vi "输入数据解析.vi"(0 "单个参数补充":dbl, 1 "从板号":dbl=1.0, 2 "主板二维码":string="BNET01", 3 "从板二维码":string="BNET01", 5 "主板引用":refnum<vi>, 7 "从板引用":refnum<vi>, 9 "主板选项":string="三级故障阀值", 11 "枚举":enum16{"主板", "从板"}(ring), 12 "快换":bool caption="快换写入") -> (4 "输出数组":dbl[][](array[numeric]), 6 "数组长度":dbl[](array[numeric]), 8 "循环次数":i32, 10 "命令":u32, 14 "名称":string[](array[string]), 15 "命令序号":u32[](array[numeric]))   [LabVIEW 2013] (continued)
                }
                n4749 = Build Array(w12371, w12369) -> (w12372:i32[])
              }
            }
            n4750 = Insert Into Array(array=w12193, new element=w12194) -> (w12192:dbl[])  [unwired: 1 in]
          }
          n4751 = Build Array(w12189) -> (w12188:dbl[][])
          n4752 = Build Array("二级故障阀值") -> (w12179:string[])
        }
        frame "SOC过低(3)" {
          n4753 = Unbundle By Name(w12398) -> ("一级故障 3"=w12399:refnum<vi>)
          n4754 = property class="Clust (严格)"(reference=w12399) -> ("Value"=w12397:T4)  [unwired: 1 in, 2 out]
          n4755 = for {
            N: 17 -> [_]
            tunnel: w12397 -> [w12409]
            shift-right: [w12406] -> w12403
            shift-left: dbl[] [] -> [w12407]
            i -> [w12410]
            n4756 = case shown="12" w12410 {
              tunnel: w12409 -> [w12411 w12422 w12433 w12443 w12453 w12463 w12475 w12487 w12499 w12511 w12523 w12535 w12547 w12559 w12566 w12575 w12584]
              tunnel: [w12412 w12423 w12434 w12444 w12454 w12465 w12477 w12489 w12501 w12513 w12525 w12536 w12549 w12561 w12565 w12574 w12586] -> w12408
              frame 0, Default {
                # "总电压过高"
                n4757 = disable-structure shown="启用" {
                  disable-tunnel: [w12418 w12421] -> w12414
                  disable-tunnel: [w12417 w12421] -> w12413
                  disable-tunnel: w12411 -> [w12416 _]
                  frame Disabled {
                    n4758 = Unbundle By Name(w12416) -> ("总电压过高"=w12415:dbl)
                    n4759 = call "输入分辨率计算-EV05.vi"("1字节?"=FALSE, "数值"=w12415, "分辨率"=0.1) -> ("低字节"=w12418:dbl, "高字节1"=w12417:dbl)  [unwired: 2 in, 5 out]
                  }
                  frame Enabled {
                    w12421 = 255 ("高字节1")
                  }
                }
                n4760 = Build Array(w12413, w12414) -> (w12412:i32[])
              }
              frame 1 {
                # "总电压过低"
                n4761 = disable-structure shown="启用" {
                  disable-tunnel: [w12429 w12432] -> w12425
                  disable-tunnel: [w12428 w12432] -> w12424
                  disable-tunnel: w12422 -> [w12427 _]
                  frame Disabled {
                    n4762 = Unbundle By Name(w12427) -> ("总电压过低"=w12426:dbl)
                    n4763 = call "输入分辨率计算-EV05.vi"("1字节?"=FALSE, "数值"=w12426, "分辨率"=0.1) -> ("低字节"=w12429:dbl, "高字节1"=w12428:dbl)  [unwired: 2 in, 5 out]
                  }
                  frame Enabled {
                    w12432 = 255 ("高字节1")
                  }
                }
                n4764 = Build Array(w12424, w12425) -> (w12423:i32[])
              }
              frame 2 {
                # "温度过高"
                n4765 = disable-structure shown="启用" {
                  disable-tunnel: [w12439 255 ("高字节1")] -> w12435
                  disable-tunnel: w12433 -> [w12437 _]
                  frame Disabled {
                    n4766 = Unbundle By Name(w12437) -> ("温度过高"=w12436:dbl)
                    n4767 = call "输入分辨率计算-EV05.vi"("1字节?"=TRUE, "数值"=w12436, "偏移量"=-40.0, "分辨率"=1.0) -> ("高字节1"=w12439:dbl)  [unwired: 1 in, 6 out]
                  }
                  frame Enabled {
                  }
                }
                n4768 = Build Array(w12435) -> (w12434:i32[])
              }
              frame 3 {
                # "温度过低"
                n4769 = disable-structure shown="启用" {
                  disable-tunnel: [w12449 255 ("高字节1")] -> w12445
                  disable-tunnel: w12443 -> [w12447 _]
                  frame Disabled {
                    n4770 = Unbundle By Name(w12447) -> ("温度过低"=w12446:dbl)
                    n4771 = call "输入分辨率计算-EV05.vi"("1字节?"=TRUE, "数值"=w12446, "偏移量"=-40.0, "分辨率"=1.0) -> ("高字节1"=w12449:dbl)  [unwired: 1 in, 6 out]
                  }
                  frame Enabled {
                  }
                }
                n4772 = Build Array(w12445) -> (w12444:i32[])
              }
              frame 4 {
                # "整组温度不均衡"
                n4773 = disable-structure shown="启用" {
                  disable-tunnel: [w12459 255 ("高字节1")] -> w12455
                  disable-tunnel: w12453 -> [w12457 _]
                  frame Disabled {
                    n4774 = Unbundle By Name(w12457) -> ("整组温度不均衡"=w12456:dbl)
                    n4775 = call "输入分辨率计算-EV05.vi"("1字节?"=TRUE, "数值"=w12456, "偏移量"=0.0, "分辨率"=1.0) -> ("高字节1"=w12459:dbl)  [unwired: 1 in, 6 out]
                  }
                  frame Enabled {
                  }
                }
                n4776 = Build Array(w12455) -> (w12454:i32[])
              }
              frame 5 {
                # "单组电压不均衡"
                n4777 = disable-structure shown="启用" {
                  disable-tunnel: [w12471 w12474] -> w12466
                  disable-tunnel: [w12469 w12474] -> w12464
                  disable-tunnel: w12463 -> [w12468 _]
                  frame Disabled {
                    n4778 = Unbundle By Name(w12468) -> ("单组电压不均衡"=w12467:dbl)
                    n4779 = call "输入分辨率计算-EV05.vi"("1字节?"=FALSE, "数值"=w12467, "偏移量"=0.0, "分辨率"=0.001) -> ("低字节"=w12469:dbl, "高字节1"=w12471:dbl)  [unwired: 1 in, 5 out]
                  }
                  frame Enabled {
                    w12474 = 255 ("高字节1")
                  }
                }
                n4780 = Build Array(w12466, w12464) -> (w12465:i32[])
              }
              frame 6 {
                # "整组电压不均衡"
                n4781 = disable-structure shown="启用" {
                  disable-tunnel: [w12483 w12486] -> w12478
                  disable-tunnel: [w12481 w12486] -> w12476
                  disable-tunnel: w12475 -> [w12480 _]
                  frame Disabled {
                    n4782 = Unbundle By Name(w12480) -> ("整组电压不均衡"=w12479:dbl)
                    n4783 = call "输入分辨率计算-EV05.vi"("1字节?"=FALSE, "数值"=w12479, "偏移量"=0.0, "分辨率"=0.001) -> ("低字节"=w12481:dbl, "高字节1"=w12483:dbl)  [unwired: 1 in, 5 out]
                  }
                  frame Enabled {
                    w12486 = 255 ("高字节1")
                  }
                }
                n4784 = Build Array(w12478, w12476) -> (w12477:i32[])
              }
              frame 7 {
                # "单体电压过高"
                n4785 = disable-structure shown="启用" {
                  disable-tunnel: [w12495 w12498] -> w12490
                  disable-tunnel: [w12493 w12498] -> w12488
                  disable-tunnel: w12487 -> [w12492 _]
                  frame Disabled {
                    n4786 = Unbundle By Name(w12492) -> ("单体电压过高"=w12491:dbl)
                    n4787 = call "输入分辨率计算-EV05.vi"("1字节?"=FALSE, "数值"=w12491, "偏移量"=0.0, "分辨率"=0.001) -> ("低字节"=w12493:dbl, "高字节1"=w12495:dbl)  [unwired: 1 in, 5 out]
                  }
                  frame Enabled {
                    w12498 = 255 ("高字节1")
                  }
                }
                n4788 = Build Array(w12490, w12488) -> (w12489:i32[])
              }
              frame 8 {
                # "单体电压过低"
                n4789 = disable-structure shown="启用" {
                  disable-tunnel: [w12507 w12510] -> w12502
                  disable-tunnel: [w12505 w12510] -> w12500
                  disable-tunnel: w12499 -> [w12504 _]
                  frame Disabled {
                    n4790 = Unbundle By Name(w12504) -> ("单体电压过低"=w12503:dbl)
                    n4791 = call "输入分辨率计算-EV05.vi"("1字节?"=FALSE, "数值"=w12503, "偏移量"=0.0, "分辨率"=0.001) -> ("低字节"=w12505:dbl, "高字节1"=w12507:dbl)  [unwired: 1 in, 5 out]
                  }
                  frame Enabled {
                    w12510 = 255 ("高字节1")
                  }
                }
                n4792 = Build Array(w12502, w12500) -> (w12501:i32[])
              }
              frame 9 {
                # "充电电流过高"
                n4793 = disable-structure shown="启用" {
                  disable-tunnel: [w12519 w12522] -> w12514
                  disable-tunnel: [w12517 w12522] -> w12512
                  disable-tunnel: w12511 -> [w12516 _]
                  frame Disabled {
                    n4794 = Unbundle By Name(w12516) -> ("充电电流过高"=w12515:dbl)
                    n4795 = call "输入分辨率计算-EV05.vi"("1字节?"=FALSE, "数值"=w12515, "偏移量"=-3000.0, "分辨率"=0.1) -> ("低字节"=w12517:dbl, "高字节1"=w12519:dbl)  [unwired: 1 in, 5 out]
                  }
                  frame Enabled {
                    w12522 = 255 ("高字节1")
                  }
                }
                n4796 = Build Array(w12514, w12512) -> (w12513:i32[])
              }
              frame 10 {
                # "放电电流过高"
                n4797 = disable-structure shown="启用" {
                  disable-tunnel: [w12531 w12534] -> w12526
                  disable-tunnel: [w12529 w12534] -> w12524
                  disable-tunnel: w12523 -> [w12528 _]
                  frame Disabled {
                    n4798 = Unbundle By Name(w12528) -> ("放电电流过高"=w12527:dbl)
                    n4799 = call "输入分辨率计算-EV05.vi"("1字节?"=FALSE, "数值"=w12527, "偏移量"=-3000.0, "分辨率"=0.1) -> ("低字节"=w12529:dbl, "高字节1"=w12531:dbl)  [unwired: 1 in, 5 out]
                  }
                  frame Enabled {
                    w12534 = 255 ("高字节1")
                  }
                }
                n4800 = Build Array(w12526, w12524) -> (w12525:i32[])
              }
              frame 11 {
                # "单组温度不均衡"
                n4801 = disable-structure shown="启用" {
                  disable-tunnel: [w12541 255 ("高字节1")] -> w12537
                  disable-tunnel: w12535 -> [w12539 _]
                  frame Disabled {
                    n4802 = Unbundle By Name(w12539) -> ("单组温度不均衡"=w12538:dbl)
                    n4803 = call "输入分辨率计算-EV05.vi"("1字节?"=TRUE, "数值"=w12538, "偏移量"=0.0, "分辨率"=1.0) -> ("高字节1"=w12541:dbl)  [unwired: 1 in, 6 out]
                  }
                  frame Enabled {
                  }
                }
                n4804 = Build Array(w12537) -> (w12536:i32[])
              }
              frame 12 {
                # "SOC过高"
                n4805 = Unbundle By Name(w12547) -> ("SOC过高"=w12546:dbl)
                n4806 = call "输入分辨率计算-EV05.vi"("1字节?"=FALSE, "数值"=w12546, "偏移量"=0.0, "分辨率"=0.1) -> ()  [unwired: 1 in, 7 out]
                n4807 = disable-structure shown="启用" {
                  disable-tunnel: _ -> [w12553 _]
                  disable-tunnel: [w12553 255 ("高字节1")] -> w12545
                  disable-tunnel: [w12552 i32[] [] ("低位子数组")] -> _
                  disable-tunnel: _ -> [w12552 _]
                  frame Disabled {
                  }
                  frame Enabled {
                  }
                }
                n4808 = Build Array(w12545, w12545) -> (w12549:i32[])
              }
              frame 13 {
                n4809 = Unbundle By Name(w12559) -> ("SOC过低"=w12558:dbl)
                n4810 = call "输入分辨率计算-EV05.vi"("1字节?"=FALSE, "数值"=w12558, "偏移量"=0.0, "分辨率"=0.1) -> ("低字节"=w12556:dbl, "高字节1"=w12557:dbl)  [unwired: 1 in, 5 out]
                n4811 = Build Array(w12557, w12556) -> (w12561:dbl[])
              }
              frame 14 {
                # "内阻过大"
                n4812 = disable-structure shown="启用" {
                  disable-tunnel: w12566 -> [w12571 _]
                  disable-tunnel: [w12567 255 ("高字节1")] -> w12564
                  frame Disabled {
                    n4813 = Unbundle By Name(w12571) -> ("内阻过大"=w12570:dbl)
                    n4814 = call "输入分辨率计算-EV05.vi"("1字节?"=TRUE, "数值"=w12570, "分辨率"=0.1) -> ("高字节1"=w12567:dbl)  [unwired: 2 in, 6 out]
                  }
                  frame Enabled {
                  }
                }
                n4815 = Build Array(w12564) -> (w12565:i32[])
              }
              frame 15 {
                # "极柱温度过高"
                n4816 = disable-structure shown="启用" {
                  disable-tunnel: w12575 -> [w12581 _]
                  disable-tunnel: [w12577 255 ("高字节1")] -> w12573
                  frame Disabled {
                    n4817 = Unbundle By Name(w12581) -> ("极柱温度过高"=w12580:dbl)
                    n4818 = call "输入分辨率计算-EV05.vi"("1字节?"=TRUE, "数值"=w12580, "偏移量"=-40.0, "分辨率"=1.0) -> ("高字节1"=w12577:dbl)  [unwired: 1 in, 6 out]
                  }
                  frame Enabled {
                  }
                }
                n4819 = Build Array(w12573) -> (w12574:i32[])
              }
              frame 16 {
                # "SOH过低"
                n4820 = disable-structure shown="启用" {
                  disable-tunnel: [w12598 w12606] -> w12585
                  disable-tunnel: w12584 -> [w12595 _]
                  disable-tunnel: [w12587 w12606] -> w12583
                  frame Disabled {
                    n4821 = Unbundle By Name(w12595) -> ("SOH过低"=w12594:dbl)
                    n4822 = call "输入分辨率计算-EV05.vi"("1字节?"=FALSE, "数值"=w12594, "偏移量"=0.0, "分辨率"=0.1) -> ("低字节"=w12596:dbl, "高字节1"=w12597:dbl)  [unwired: 1 in, 5 out]
                    n4823 = call "二进制解析-8.6.vi"("索引"=4, "数值"=w12597) -> ("低位子数组"=w12600:i32[])  [unwired: 3 out]
                    n4824 = call "二进制解析-8.6.vi"("索引"=4, "数值"=w12596) -> ("低位子数组"=w12589:i32[], "高位子数组"=w12599:i32[])  [unwired: 2 out]
                    n4825 = call "二进制解析-8.6.vi"("索引"=4, "数值"=0) -> ("低位子数组"=w12590:i32[])  [unwired: 3 out]
                    n4826 = Insert Into Array(array=w12600, new element=w12599) -> (w12593:i32[])  [unwired: 1 in]
                    n4827 = Insert Into Array(array=w12589, new element=w12590) -> (w12588:i32[])  [unwired: 1 in]
                    n4828 = call "数值二进制转十进制-8.6.vi"("子数组"=w12593) -> ("十进制数值"=w12598:i32)  [unwired: 4 out]
                    n4829 = call "数值二进制转十进制-8.6.vi"("子数组"=w12588) -> ("十进制数值"=w12587:i32)  [unwired: 4 out]
                  }
                  frame Enabled {
                    w12606 = 255 ("高字节1")
                  }
                }
                n4830 = Build Array(w12585, w12583) -> (w12586:i32[])
              }
            }
            n4831 = Insert Into Array(array=w12407, new element=w12408) -> (w12406:dbl[])  [unwired: 1 in]
          }
          n4832 = Build Array(w12403) -> (w12402:dbl[][])
          n4833 = Build Array("三级故障阀值") -> (w12393:string[])
        }
        frame "二级故障阀值" {
          n4834 = Unbundle By Name(w12612) -> ("一级故障 2"=w12613:refnum<vi>)
          n4835 = property class="Clust (严格)"(reference=w12613) -> ("Value"=w12611:T4)  [unwired: 1 in, 2 out]
          n4836 = for {
            N: 17 -> [_]
            tunnel: w12611 -> [w12623]
            shift-right: [w12620] -> w12617
            shift-left: dbl[] [] -> [w12621]
            i -> [w12624]
            n4837 = case shown="4" w12624 {
              tunnel: w12623 -> [w12626 w12633 w12640 w12647 w12654 w12660 w12668 w12676 w12684 w12692 w12700 w12708 w12716 w12724 w12734 w12741 w12745]
              tunnel: [w12627 w12634 w12642 w12649 w12655 w12663 w12671 w12679 w12687 w12695 w12703 w12709 w12718 w12726 w12733 w12740 w12747] -> w12622
              frame 0, Default {
                # "总电压过高"
                n4838 = Unbundle By Name(w12626) -> ("总电压过高"=w12625:dbl)
                n4839 = call "输入分辨率计算-EV05.vi"("1字节?"=FALSE, "数值"=w12625, "分辨率"=0.1) -> ("低字节"=w12629:dbl, "高字节1"=w12628:dbl)  [unwired: 2 in, 5 out]
                n4840 = Build Array(w12628, w12629) -> (w12627:dbl[])
              }
              frame 1 {
                # "总电压过低"
                n4841 = Unbundle By Name(w12633) -> ("总电压过低"=w12632:dbl)
                n4842 = call "输入分辨率计算-EV05.vi"("1字节?"=FALSE, "数值"=w12632, "分辨率"=0.1) -> ("低字节"=w12636:dbl, "高字节1"=w12635:dbl)  [unwired: 2 in, 5 out]
                n4843 = Build Array(w12635, w12636) -> (w12634:dbl[])
              }
              frame 2 {
                # "温度过高"
                n4844 = Unbundle By Name(w12640) -> ("温度过高"=w12639:dbl)
                n4845 = call "输入分辨率计算-EV05.vi"("1字节?"=TRUE, "数值"=w12639, "偏移量"=-40.0, "分辨率"=1.0) -> ("高字节1"=w12643:dbl)  [unwired: 1 in, 6 out]
                n4846 = Build Array(w12643) -> (w12642:dbl[])
              }
              frame 3 {
                # "温度过低"
                n4847 = Unbundle By Name(w12647) -> ("温度过低"=w12646:dbl)
                n4848 = call "输入分辨率计算-EV05.vi"("1字节?"=TRUE, "数值"=w12646, "偏移量"=-40.0, "分辨率"=1.0) -> ("高字节1"=w12650:dbl)  [unwired: 1 in, 6 out]
                n4849 = Build Array(w12650) -> (w12649:dbl[])
              }
              frame 4 {
                # "整组温度不均衡"
                n4850 = Unbundle By Name(w12654) -> ("整组温度不均衡"=w12653:dbl)
                n4851 = call "输入分辨率计算-EV05.vi"("1字节?"=TRUE, "数值"=w12653, "分辨率"=1.0) -> ("高字节1"=w12656:dbl)  [unwired: 2 in, 6 out]
                n4852 = Build Array(w12656) -> (w12655:dbl[])
              }
              frame 5 {
                # "单组电压不均衡"
                n4853 = Unbundle By Name(w12660) -> ("单组电压不均衡"=w12659:dbl)
                n4854 = call "输入分辨率计算-EV05.vi"("1字节?"=FALSE, "数值"=w12659, "偏移量"=0.0, "分辨率"=0.001) -> ("低字节"=w12661:dbl, "高字节1"=w12664:dbl)  [unwired: 1 in, 5 out]
                n4855 = Build Array(w12664, w12661) -> (w12663:dbl[])
              }
              frame 6 {
                # "整组电压不均衡"
                n4856 = Unbundle By Name(w12668) -> ("整组电压不均衡"=w12667:dbl)
                n4857 = call "输入分辨率计算-EV05.vi"("1字节?"=FALSE, "数值"=w12667, "偏移量"=0.0, "分辨率"=0.001) -> ("低字节"=w12669:dbl, "高字节1"=w12672:dbl)  [unwired: 1 in, 5 out]
                n4858 = Build Array(w12672, w12669) -> (w12671:dbl[])
              }
              frame 7 {
                # "单体电压过高"
                n4859 = Unbundle By Name(w12676) -> ("单体电压过高"=w12675:dbl)
                n4860 = call "输入分辨率计算-EV05.vi"("1字节?"=FALSE, "数值"=w12675, "偏移量"=0.0, "分辨率"=0.001) -> ("低字节"=w12677:dbl, "高字节1"=w12680:dbl)  [unwired: 1 in, 5 out]
                n4861 = Build Array(w12680, w12677) -> (w12679:dbl[])
              }
              frame 8 {
                # "单体电压过低"
                n4862 = Unbundle By Name(w12684) -> ("单体电压过低"=w12683:dbl)
                n4863 = call "输入分辨率计算-EV05.vi"("1字节?"=FALSE, "数值"=w12683, "偏移量"=0.0, "分辨率"=0.001) -> ("低字节"=w12685:dbl, "高字节1"=w12688:dbl)  [unwired: 1 in, 5 out]
                n4864 = Build Array(w12688, w12685) -> (w12687:dbl[])
              }
              frame 9 {
                # "充电电流过高"
                n4865 = Unbundle By Name(w12692) -> ("充电电流过高"=w12691:dbl)
                n4866 = call "输入分辨率计算-EV05.vi"("1字节?"=FALSE, "数值"=w12691, "偏移量"=0.0, "分辨率"=0.1) -> ("低字节"=w12693:dbl, "高字节1"=w12696:dbl)  [unwired: 1 in, 5 out]
                n4867 = Build Array(w12696, w12693) -> (w12695:dbl[])
              }
              frame 10 {
                # "放电电流过高"
                n4868 = Unbundle By Name(w12700) -> ("放电电流过高"=w12699:dbl)
                n4869 = call "输入分辨率计算-EV05.vi"("1字节?"=FALSE, "数值"=w12699, "偏移量"=0.0, "分辨率"=0.1) -> ("低字节"=w12701:dbl, "高字节1"=w12704:dbl)  [unwired: 1 in, 5 out]
                n4870 = Build Array(w12704, w12701) -> (w12703:dbl[])
              }
              frame 11 {
                # "单组温度不均衡"
                n4871 = Unbundle By Name(w12708) -> ("单组温度不均衡"=w12707:dbl)
                n4872 = call "输入分辨率计算-EV05.vi"("1字节?"=TRUE, "数值"=w12707, "分辨率"=1.0) -> ("高字节1"=w12710:dbl)  [unwired: 2 in, 6 out]
                n4873 = Build Array(w12710) -> (w12709:dbl[])
              }
              frame 12 {
                # "SOC过高"
                n4874 = Unbundle By Name(w12716) -> ("SOC过高"=w12715:dbl)
                n4875 = call "输入分辨率计算-EV05.vi"("1字节?"=FALSE, "数值"=w12715, "偏移量"=0.0, "分辨率"=0.1) -> ("低字节"=w12713:dbl, "高字节1"=w12714:dbl)  [unwired: 1 in, 5 out]
                n4876 = Build Array(w12714, w12713) -> (w12718:dbl[])
              }
              frame 13 {
                # "SOC过低"
                n4877 = Unbundle By Name(w12724) -> ("SOC过低"=w12723:dbl)
                n4878 = call "输入分辨率计算-EV05.vi"("1字节?"=FALSE, "数值"=w12723, "偏移量"=0.0, "分辨率"=0.1) -> ("低字节"=w12721:dbl, "高字节1"=w12722:dbl)  [unwired: 1 in, 5 out]
                n4879 = Build Array(w12722, w12721) -> (w12726:dbl[])
              }
              frame 14 {
                # "内阻过大"
                n4880 = Unbundle By Name(w12734) -> ("内阻过大"=w12732:dbl)
                n4881 = call "输入分辨率计算-EV05.vi"("1字节?"=TRUE, "数值"=w12732, "分辨率"=0.1) -> ("高字节1"=w12729:dbl)  [unwired: 2 in, 6 out]
                n4882 = Build Array(w12729) -> (w12733:dbl[])
              }
              frame 15 {
                # "极柱温度过高"
                n4883 = Unbundle By Name(w12741) -> ("极柱温度过高"=w12739:dbl)
                n4884 = call "输入分辨率计算-EV05.vi"("1字节?"=TRUE, "数值"=w12739, "偏移量"=-40.0, "分辨率"=1.0) -> ("高字节1"=w12736:dbl)  [unwired: 1 in, 6 out]
                n4885 = Build Array(w12736) -> (w12740:dbl[])
              }
              frame 16 {
                # "SOH过低"
                n4886 = Unbundle By Name(w12745) -> ("SOH过低"=w12744:dbl)
                n4887 = call "输入分辨率计算-EV05.vi"("1字节?"=FALSE, "数值"=w12744, "偏移量"=0.0, "分辨率"=0.1) -> ("低字节"=w12742:dbl, "高字节1"=w12743:dbl)  [unwired: 1 in, 5 out]
                n4888 = Build Array(w12743, w12742) -> (w12747:dbl[])
              }
            }
            n4889 = Insert Into Array(array=w12621, new element=w12622) -> (w12620:dbl[])  [unwired: 1 in]
          }
          n4890 = Build Array(w12617) -> (w12616:dbl[][])
          n4891 = Build Array("二级故障阀值") -> (w12607:string[])
        }
        frame "三级故障阀值" {
          n4892 = Unbundle By Name(w12755) -> ("一级故障 3"=w12756:refnum<vi>)
          n4893 = property class="Clust (严格)"(reference=w12756) -> ("Value"=w12754:T4)  [unwired: 1 in, 2 out]
          n4894 = for {
            N: 17 -> [_]
            tunnel: w12754 -> [w12766]
            shift-right: [w12763] -> w12760
            shift-left: dbl[] [] -> [w12764]
            i -> [w12767]
            n4895 = case shown="11" w12767 {
              tunnel: w12766 -> [w12769 w12776 w12783 w12790 w12797 w12803 w12811 w12819 w12827 w12835 w12843 w12851 w12859 w12867 w12877 w12884 w12888]
              tunnel: [w12770 w12777 w12785 w12792 w12798 w12806 w12814 w12822 w12830 w12838 w12846 w12852 w12861 w12869 w12876 w12883 w12890] -> w12765
              frame 0, Default {
                # "总电压过高"
                n4896 = Unbundle By Name(w12769) -> ("总电压过高"=w12768:dbl)
                n4897 = call "输入分辨率计算-EV05.vi"("1字节?"=FALSE, "数值"=w12768, "分辨率"=0.1) -> ("低字节"=w12772:dbl, "高字节1"=w12771:dbl)  [unwired: 2 in, 5 out]
                n4898 = Build Array(w12771, w12772) -> (w12770:dbl[])
              }
              frame 1 {
                # "总电压过低"
                n4899 = Unbundle By Name(w12776) -> ("总电压过低"=w12775:dbl)
                n4900 = call "输入分辨率计算-EV05.vi"("1字节?"=FALSE, "数值"=w12775, "分辨率"=0.1) -> ("低字节"=w12779:dbl, "高字节1"=w12778:dbl)  [unwired: 2 in, 5 out]
                n4901 = Build Array(w12778, w12779) -> (w12777:dbl[])
              }
              frame 2 {
                # "温度过高"
                n4902 = Unbundle By Name(w12783) -> ("温度过高"=w12782:dbl)
                n4903 = call "输入分辨率计算-EV05.vi"("1字节?"=TRUE, "数值"=w12782, "偏移量"=-40.0, "分辨率"=1.0) -> ("高字节1"=w12786:dbl)  [unwired: 1 in, 6 out]
                n4904 = Build Array(w12786) -> (w12785:dbl[])
              }
              frame 3 {
                # "温度过低"
                n4905 = Unbundle By Name(w12790) -> ("温度过低"=w12789:dbl)
                n4906 = call "输入分辨率计算-EV05.vi"("1字节?"=TRUE, "数值"=w12789, "偏移量"=-40.0, "分辨率"=1.0) -> ("高字节1"=w12793:dbl)  [unwired: 1 in, 6 out]
                n4907 = Build Array(w12793) -> (w12792:dbl[])
              }
              frame 4 {
                # "整组温度不均衡"
                n4908 = Unbundle By Name(w12797) -> ("整组温度不均衡"=w12796:dbl)
                n4909 = call "输入分辨率计算-EV05.vi"("1字节?"=TRUE, "数值"=w12796, "分辨率"=1.0) -> ("高字节1"=w12799:dbl)  [unwired: 2 in, 6 out]
                n4910 = Build Array(w12799) -> (w12798:dbl[])
              }
              frame 5 {
                # "单组电压不均衡"
                n4911 = Unbundle By Name(w12803) -> ("单组电压不均衡"=w12802:dbl)
                n4912 = call "输入分辨率计算-EV05.vi"("1字节?"=FALSE, "数值"=w12802, "偏移量"=0.0, "分辨率"=0.001) -> ("低字节"=w12804:dbl, "高字节1"=w12807:dbl)  [unwired: 1 in, 5 out]
                n4913 = Build Array(w12807, w12804) -> (w12806:dbl[])
              }
              frame 6 {
                # "整组电压不均衡"
                n4914 = Unbundle By Name(w12811) -> ("整组电压不均衡"=w12810:dbl)
                n4915 = call "输入分辨率计算-EV05.vi"("1字节?"=FALSE, "数值"=w12810, "偏移量"=0.0, "分辨率"=0.001) -> ("低字节"=w12812:dbl, "高字节1"=w12815:dbl)  [unwired: 1 in, 5 out]
                n4916 = Build Array(w12815, w12812) -> (w12814:dbl[])
              }
              frame 7 {
                # "单体电压过高"
                n4917 = Unbundle By Name(w12819) -> ("单体电压过高"=w12818:dbl)
                n4918 = call "输入分辨率计算-EV05.vi"("1字节?"=FALSE, "数值"=w12818, "偏移量"=0.0, "分辨率"=0.001) -> ("低字节"=w12820:dbl, "高字节1"=w12823:dbl)  [unwired: 1 in, 5 out]
                n4919 = Build Array(w12823, w12820) -> (w12822:dbl[])
              }
              frame 8 {
                # "单体电压过低"
                n4920 = Unbundle By Name(w12827) -> ("单体电压过低"=w12826:dbl)
                n4921 = call "输入分辨率计算-EV05.vi"("1字节?"=FALSE, "数值"=w12826, "偏移量"=0.0, "分辨率"=0.001) -> ("低字节"=w12828:dbl, "高字节1"=w12831:dbl)  [unwired: 1 in, 5 out]
                n4922 = Build Array(w12831, w12828) -> (w12830:dbl[])
              }
              frame 9 {
                # "充电电流过高"
                n4923 = Unbundle By Name(w12835) -> ("充电电流过高"=w12834:dbl)
                n4924 = call "输入分辨率计算-EV05.vi"("1字节?"=FALSE, "数值"=w12834, "偏移量"=0.0, "分辨率"=0.1) -> ("低字节"=w12836:dbl, "高字节1"=w12839:dbl)  [unwired: 1 in, 5 out]
                n4925 = Build Array(w12839, w12836) -> (w12838:dbl[])
              }
              frame 10 {
                # "放电电流过高"
                n4926 = Unbundle By Name(w12843) -> ("放电电流过高"=w12842:dbl)
                n4927 = call "输入分辨率计算-EV05.vi"("1字节?"=FALSE, "数值"=w12842, "偏移量"=0.0, "分辨率"=0.1) -> ("低字节"=w12844:dbl, "高字节1"=w12847:dbl)  [unwired: 1 in, 5 out]
                n4928 = Build Array(w12847, w12844) -> (w12846:dbl[])
              }
              frame 11 {
                # "单组温度不均衡"
                n4929 = Unbundle By Name(w12851) -> ("单组温度不均衡"=w12850:dbl)
                n4930 = call "输入分辨率计算-EV05.vi"("1字节?"=TRUE, "数值"=w12850, "分辨率"=1.0) -> ("高字节1"=w12853:dbl)  [unwired: 2 in, 6 out]
                n4931 = Build Array(w12853) -> (w12852:dbl[])
              }
              frame 12 {
                # "SOC过高"
                n4932 = Unbundle By Name(w12859) -> ("SOC过高"=w12858:dbl)
                n4933 = call "输入分辨率计算-EV05.vi"("1字节?"=FALSE, "数值"=w12858, "偏移量"=0.0, "分辨率"=0.1) -> ("低字节"=w12856:dbl, "高字节1"=w12857:dbl)  [unwired: 1 in, 5 out]
                n4934 = Build Array(w12857, w12856) -> (w12861:dbl[])
              }
              frame 13 {
                # "SOC过低"
                n4935 = Unbundle By Name(w12867) -> ("SOC过低"=w12866:dbl)
                n4936 = call "输入分辨率计算-EV05.vi"("1字节?"=FALSE, "数值"=w12866, "偏移量"=0.0, "分辨率"=0.1) -> ("低字节"=w12864:dbl, "高字节1"=w12865:dbl)  [unwired: 1 in, 5 out]
                n4937 = Build Array(w12865, w12864) -> (w12869:dbl[])
              }
              frame 14 {
                # "内阻过大"
                n4938 = Unbundle By Name(w12877) -> ("内阻过大"=w12875:dbl)
                n4939 = call "输入分辨率计算-EV05.vi"("1字节?"=TRUE, "数值"=w12875, "分辨率"=0.1) -> ("高字节1"=w12872:dbl)  [unwired: 2 in, 6 out]
                n4940 = Build Array(w12872) -> (w12876:dbl[])
              }
              frame 15 {
                # "极柱温度过高"
                n4941 = Unbundle By Name(w12884) -> ("极柱温度过高"=w12882:dbl)
                n4942 = call "输入分辨率计算-EV05.vi"("1字节?"=TRUE, "数值"=w12882, "偏移量"=-40.0, "分辨率"=1.0) -> ("高字节1"=w12879:dbl)  [unwired: 1 in, 6 out]
                n4943 = Build Array(w12879) -> (w12883:dbl[])
              }
              frame 16 {
                # "SOH过低"
                n4944 = Unbundle By Name(w12888) -> ("SOH过低"=w12887:dbl)
                n4945 = call "输入分辨率计算-EV05.vi"("1字节?"=FALSE, "数值"=w12887, "偏移量"=0.0, "分辨率"=0.1) -> ("低字节"=w12885:dbl, "高字节1"=w12886:dbl)  [unwired: 1 in, 5 out]
                n4946 = Build Array(w12886, w12885) -> (w12890:dbl[])
              }
            }
            n4947 = Insert Into Array(array=w12764, new element=w12765) -> (w12763:dbl[])  [unwired: 1 in]
          }
          n4948 = Build Array(w12760) -> (w12759:dbl[][])
          n4949 = Build Array("三级故障阀值") -> (w12750:string[])
        }
        frame "加热控制参数" {
          n4950 = Unbundle By Name(w12914) -> ("加热控制参数"=w12915:refnum<vi>)
          n4951 = property class="Clust (严格)"(reference=w12915) -> ("Value"=w12913:T5)  [unwired: 1 in, 2 out]
          n4952 = Unbundle(w12913) -> ("风机开启温度"=w12908:dbl, "风机关闭温度"=w12907:dbl, "加热开启温度"=w12904:dbl, "加热关闭温度"=w12903:dbl, "风机开启温差"=w12897:dbl, "风机关闭温差"=w12896:dbl, "加热关闭温差"=w12893:dbl)
          n4953 = call "输入分辨率计算-EV05.vi"("1字节?"=TRUE, "数值 2"=w12903, "数值"=w12904, "偏移量"=-40.0, "分辨率"=1.0) -> ("高字节 2"=w12894:dbl, "高字节1"=w12895:dbl)  [unwired: 5 out]
          n4954 = call "输入分辨率计算-EV05.vi"("1字节?"=TRUE, "数值 2"=w12907, "数值"=w12908, "偏移量"=-40.0, "分辨率"=1.0) -> ("高字节 2"=w12901:dbl, "高字节1"=w12902:dbl)  [unwired: 5 out]
          n4955 = Build Array(w12902, w12901, w12897, w12896, w12895, w12894, w12893) -> (w12900:dbl[])
          n4956 = Build Array(w12900) -> (w12918:dbl[][])
        }
        frame "风机开启温度" {
          w12920 = 255 ("高字节1")
          n4957 = Unbundle By Name(w12936) -> ("加热控制参数"=w12937:refnum<vi>)
          n4958 = property class="Clust (严格)"(reference=w12937) -> ("Value"=w12935:T5)  [unwired: 1 in, 2 out]
          n4959 = Unbundle(w12935) -> ("风机开启温度"=w12930:dbl, "风机关闭温度"=w12929:dbl, "加热开启温度"=w12926:dbl, "加热关闭温度"=w12925:dbl)  [unwired: 3 out]
          n4960 = call "输入分辨率计算-EV05.vi"("1字节?"=TRUE, "数值 2"=w12925, "数值"=w12926, "偏移量"=-40.0, "分辨率"=1.0) -> ()  [unwired: 7 out]
          n4961 = call "输入分辨率计算-EV05.vi"("1字节?"=TRUE, "数值 2"=w12929, "数值"=w12930, "偏移量"=-40.0, "分辨率"=1.0) -> ("高字节1"=w12924:dbl)  [unwired: 6 out]
          n4962 = Build Array(w12924, w12920, w12920, w12920, w12920, w12920, w12920) -> (w12923:dbl[])
          n4963 = Build Array(w12923) -> (w12940:dbl[][])
        }
        frame "风机关闭温度" {
          w12942 = 255 ("高字节1")
          n4964 = Unbundle By Name(w12958) -> ("加热控制参数"=w12959:refnum<vi>)
          n4965 = property class="Clust (严格)"(reference=w12959) -> ("Value"=w12957:T5)  [unwired: 1 in, 2 out]
          n4966 = Unbundle(w12957) -> ("风机开启温度"=w12952:dbl, "风机关闭温度"=w12951:dbl, "加热开启温度"=w12948:dbl, "加热关闭温度"=w12947:dbl)  [unwired: 3 out]
          n4967 = call "输入分辨率计算-EV05.vi"("1字节?"=TRUE, "数值 2"=w12947, "数值"=w12948, "偏移量"=-40.0, "分辨率"=1.0) -> ()  [unwired: 7 out]
          n4968 = call "输入分辨率计算-EV05.vi"("1字节?"=TRUE, "数值 2"=w12951, "数值"=w12952, "偏移量"=-40.0, "分辨率"=1.0) -> ("高字节 2"=w12945:dbl)  [unwired: 6 out]
          n4969 = Build Array(w12942, w12945, w12942, w12942, w12942, w12942, w12942) -> (w12946:dbl[])
          n4970 = Build Array(w12946) -> (w12962:dbl[][])
        }
        frame "加热开启温度" {
          w12964 = 255 ("高字节1")
          n4971 = Unbundle By Name(w12980) -> ("加热控制参数"=w12981:refnum<vi>)
          n4972 = property class="Clust (严格)"(reference=w12981) -> ("Value"=w12979:T5)  [unwired: 1 in, 2 out]
          n4973 = Unbundle(w12979) -> ("风机开启温度"=w12974:dbl, "风机关闭温度"=w12973:dbl, "加热开启温度"=w12970:dbl, "加热关闭温度"=w12969:dbl)  [unwired: 3 out]
          n4974 = call "输入分辨率计算-EV05.vi"("1字节?"=TRUE, "数值 2"=w12969, "数值"=w12970, "偏移量"=-40.0, "分辨率"=1.0) -> ("高字节1"=w12965:dbl)  [unwired: 6 out]
          n4975 = call "输入分辨率计算-EV05.vi"("1字节?"=TRUE, "数值 2"=w12973, "数值"=w12974, "偏移量"=-40.0, "分辨率"=1.0) -> ()  [unwired: 7 out]
          n4976 = Build Array(w12964, w12964, w12964, w12964, w12965, w12964, w12964) -> (w12968:dbl[])
          n4977 = Build Array(w12968) -> (w12984:dbl[][])
        }
        frame "加热关闭温度" {
          w12986 = 255 ("高字节1")
          n4978 = Unbundle By Name(w13002) -> ("加热控制参数"=w13003:refnum<vi>)
          n4979 = property class="Clust (严格)"(reference=w13003) -> ("Value"=w13001:T5)  [unwired: 1 in, 2 out]
          n4980 = Unbundle(w13001) -> ("风机开启温度"=w12996:dbl, "风机关闭温度"=w12995:dbl, "加热开启温度"=w12992:dbl, "加热关闭温度"=w12991:dbl)  [unwired: 3 out]
          n4981 = call "输入分辨率计算-EV05.vi"("1字节?"=TRUE, "数值 2"=w12991, "数值"=w12992, "偏移量"=-40.0, "分辨率"=1.0) -> ("高字节 2"=w12987:dbl)  [unwired: 6 out]
          n4982 = call "输入分辨率计算-EV05.vi"("1字节?"=TRUE, "数值 2"=w12995, "数值"=w12996, "偏移量"=-40.0, "分辨率"=1.0) -> ()  [unwired: 7 out]
          n4983 = Build Array(w12986, w12986, w12986, w12986, w12986, w12987, w12986) -> (w12990:dbl[])
          n4984 = Build Array(w12990) -> (w13006:dbl[][])
        }
        frame "风机开启温差" {
          w13008 = 255 ("高字节1")
          n4985 = Unbundle By Name(w13024) -> ("加热控制参数"=w13025:refnum<vi>)
          n4986 = property class="Clust (严格)"(reference=w13025) -> ("Value"=w13023:T5)  [unwired: 1 in, 2 out]
          n4987 = Unbundle(w13023) -> ("风机开启温度"=w13018:dbl, "风机关闭温度"=w13017:dbl, "加热开启温度"=w13014:dbl, "加热关闭温度"=w13013:dbl, "风机开启温差"=w13009:dbl)  [unwired: 2 out]
          n4988 = call "输入分辨率计算-EV05.vi"("1字节?"=TRUE, "数值 2"=w13013, "数值"=w13014, "偏移量"=-40.0, "分辨率"=1.0) -> ()  [unwired: 7 out]
          n4989 = call "输入分辨率计算-EV05.vi"("1字节?"=TRUE, "数值 2"=w13017, "数值"=w13018, "偏移量"=-40.0, "分辨率"=1.0) -> ()  [unwired: 7 out]
          n4990 = Build Array(w13008, w13008, w13009, w13008, w13008, w13008, w13008) -> (w13012:dbl[])
          n4991 = Build Array(w13012) -> (w13028:dbl[][])
        }
        frame "风机关闭温差" {
          w13030 = 255 ("高字节1")
          n4992 = Unbundle By Name(w13046) -> ("加热控制参数"=w13047:refnum<vi>)
          n4993 = property class="Clust (严格)"(reference=w13047) -> ("Value"=w13045:T5)  [unwired: 1 in, 2 out]
          n4994 = Unbundle(w13045) -> ("风机开启温度"=w13040:dbl, "风机关闭温度"=w13039:dbl, "加热开启温度"=w13036:dbl, "加热关闭温度"=w13035:dbl, "风机关闭温差"=w13031:dbl)  [unwired: 2 out]
          n4995 = call "输入分辨率计算-EV05.vi"("1字节?"=TRUE, "数值 2"=w13035, "数值"=w13036, "偏移量"=-40.0, "分辨率"=1.0) -> ()  [unwired: 7 out]
          n4996 = call "输入分辨率计算-EV05.vi"("1字节?"=TRUE, "数值 2"=w13039, "数值"=w13040, "偏移量"=-40.0, "分辨率"=1.0) -> ()  [unwired: 7 out]
          n4997 = Build Array(w13030, w13030, w13030, w13031, w13030, w13030, w13030) -> (w13034:dbl[])
          n4998 = Build Array(w13034) -> (w13050:dbl[][])
        }
        frame "加热关闭温差" {
          w13053 = 255 ("高字节1")
          n4999 = Unbundle By Name(w13068) -> ("加热控制参数"=w13069:refnum<vi>)
          n5000 = property class="Clust (严格)"(reference=w13069) -> ("Value"=w13067:T5)  [unwired: 1 in, 2 out]
          n5001 = Unbundle(w13067) -> ("风机开启温度"=w13062:dbl, "风机关闭温度"=w13061:dbl, "加热开启温度"=w13058:dbl, "加热关闭温度"=w13057:dbl, "加热关闭温差"=w13052:dbl)  [unwired: 2 out]
          n5002 = call "输入分辨率计算-EV05.vi"("1字节?"=TRUE, "数值 2"=w13057, "数值"=w13058, "偏移量"=-40.0, "分辨率"=1.0) -> ()  [unwired: 7 out]
          n5003 = call "输入分辨率计算-EV05.vi"("1字节?"=TRUE, "数值 2"=w13061, "数值"=w13062, "偏移量"=-40.0, "分辨率"=1.0) -> ()  [unwired: 7 out]
          n5004 = Build Array(w13053, w13053, w13053, w13053, w13053, w13053, w13052) -> (w13056:dbl[])
          n5005 = Build Array(w13056) -> (w13072:dbl[][])
        }
        frame "充电控制参数" {
          n5006 = Unbundle By Name(w13077) -> ("充电控制参数"=w13078:refnum<vi>)
          n5007 = property class="Clust (严格)"(reference=w13078) -> ("Value"=w13076:T6)  [unwired: 1 in, 2 out]
          n5008 = for {
            N: 8 -> [_]
            tunnel: w13076 -> [w13088]
            shift-right: [w13090] -> w13082
            shift-left: dbl[] [] -> [w13086]
            i -> [w13089]
            n5009 = case shown="5" w13089 {
              tunnel: w13088 -> [w13092 w13099 w13106 w13114 w13121 w13128 w13136 w13143]
              tunnel: [w13093 w13100 w13108 w13116 w13123 w13131 w13138 w13145] -> w13087
              frame 0, Default {
                # "最大允许单体电压"
                n5010 = Unbundle By Name(w13092) -> ("最大允许单体电压"=w13091:dbl)
                n5011 = call "输入分辨率计算-EV05.vi"("1字节?"=FALSE, "数值"=w13091, "分辨率"=0.001) -> ("低字节"=w13094:dbl, "高字节1"=w13095:dbl)  [unwired: 2 in, 5 out]
                n5012 = Build Array(w13095, w13094) -> (w13093:dbl[])
              }
              frame 1 {
                # "最大允许总电压"
                n5013 = Unbundle By Name(w13099) -> ("最大允许总电压"=w13098:dbl)
                n5014 = call "输入分辨率计算-EV05.vi"("1字节?"=FALSE, "数值"=w13098, "分辨率"=0.1) -> ("低字节"=w13101:dbl, "高字节1"=w13102:dbl)  [unwired: 2 in, 5 out]
                n5015 = Build Array(w13102, w13101) -> (w13100:dbl[])
              }
              frame 2 {
                # "最大允许充电电流"
                n5016 = Unbundle By Name(w13106) -> ("最大允许充电电流"=w13105:dbl)
                n5017 = call "输入分辨率计算-EV05.vi"("1字节?"=FALSE, "数值"=w13105, "偏移量"=0.0, "分辨率"=0.1) -> ("低字节"=w13109:dbl, "高字节1"=w13110:dbl)  [unwired: 1 in, 5 out]
                n5018 = Build Array(w13110, w13109) -> (w13108:dbl[])
              }
              frame 3 {
                # "最小允许充电温度"
                n5019 = Unbundle By Name(w13114) -> ("最小允许充电温度"=w13113:dbl)
                n5020 = call "输入分辨率计算-EV05.vi"("1字节?"=TRUE, "数值"=w13113, "偏移量"=-40.0, "分辨率"=1.0) -> ("高字节1"=w13117:dbl)  [unwired: 1 in, 6 out]
                n5021 = Build Array(w13117) -> (w13116:dbl[])
              }
              frame 4 {
                # "最小充电电流"
                n5022 = Unbundle By Name(w13121) -> ("最小允许充电电流"=w13120:dbl)
                n5023 = call "输入分辨率计算-EV05.vi"("1字节?"=FALSE, "数值"=w13120, "分辨率"=0.1) -> ("低字节"=w13122:dbl, "高字节1"=w13124:dbl)  [unwired: 2 in, 5 out]
                n5024 = Build Array(w13124, w13122) -> (w13123:dbl[])
              }
              frame 5 {
                # "电流步长"
                n5025 = Unbundle By Name(w13128) -> ("电流步长"=w13127:dbl)
                n5026 = call "输入分辨率计算-EV05.vi"("1字节?"=FALSE, "数值"=w13127, "偏移量"=0.0, "分辨率"=0.1) -> ("低字节"=w13129:dbl, "高字节1"=w13132:dbl)  [unwired: 1 in, 5 out]
                n5027 = Build Array(w13132, w13129) -> (w13131:dbl[])
              }
              frame 6 {
                # "最小允许单体电压"
                n5028 = Unbundle By Name(w13136) -> ("最小允许单体电压"=w13135:dbl)
                n5029 = call "输入分辨率计算-EV05.vi"("1字节?"=FALSE, "数值"=w13135, "分辨率"=0.001) -> ("低字节"=w13137:dbl, "高字节1"=w13139:dbl)  [unwired: 2 in, 5 out]
                n5030 = Build Array(w13139, w13137) -> (w13138:dbl[])
              }
              frame 7 {
                # "最大允许充电温度"
                n5031 = Unbundle By Name(w13143) -> ("最大允许充电温度"=w13142:dbl)
                n5032 = call "输入分辨率计算-EV05.vi"("1字节?"=TRUE, "数值"=w13142, "偏移量"=-40.0, "分辨率"=1.0) -> ("高字节1"=w13146:dbl)  [unwired: 1 in, 6 out]
                n5033 = Build Array(w13146) -> (w13145:dbl[])
              }
            }
            n5034 = Insert Into Array(array=w13086, new element=w13087) -> (w13090:dbl[])  [unwired: 1 in]
          }
          n5035 = Build Array(w13082) -> (w13084:dbl[][])
        }
        frame "最大允许单体电压" {
          n5036 = Unbundle By Name(w13152) -> ("充电控制参数"=w13153:refnum<vi>)
          n5037 = property class="Clust (严格)"(reference=w13153) -> ("Value"=w13151:T6)  [unwired: 1 in, 2 out]
          n5038 = for {
            N: 8 -> [_]
            tunnel: w13151 -> [w13163]
            shift-right: [w13165] -> w13157
            shift-left: dbl[] [] -> [w13161]
            i -> [w13164]
            n5039 = case shown="0, 默认" w13164 {
              tunnel: w13163 -> [w13166 w13177 w13188 w13200 w13210 w13221 w13233 w13244]
              tunnel: [w13167 w13178 w13189 w13201 w13212 w13223 w13235 w13245] -> w13162
              frame 0, Default {
                # "最大允许单体电压"
                n5040 = disable-structure shown="启用" {
                  disable-tunnel: [w13173 w13176] -> w13169
                  disable-tunnel: [w13172 w13176] -> w13168
                  disable-tunnel: w13166 -> [w13171 _]
                  frame Enabled {
                    n5041 = Unbundle By Name(w13171) -> ("最大允许单体电压"=w13170:dbl)
                    n5042 = call "输入分辨率计算-EV05.vi"("1字节?"=FALSE, "数值"=w13170, "分辨率"=0.001) -> ("低字节"=w13172:dbl, "高字节1"=w13173:dbl)  [unwired: 2 in, 5 out]
                  }
                  frame Disabled {
                    w13176 = 255 ("高字节1")
                  }
                }
                n5043 = Build Array(w13169, w13168) -> (w13167:dbl[])
              }
              frame 1 {
                # "最大允许总电压"
                n5044 = disable-structure shown="启用" {
                  disable-tunnel: [w13184 w13187] -> w13180
                  disable-tunnel: [w13183 w13187] -> w13179
                  disable-tunnel: w13177 -> [w13182 _]
                  frame Disabled {
                    n5045 = Unbundle By Name(w13182) -> ("最大允许总电压"=w13181:dbl)
                    n5046 = call "输入分辨率计算-EV05.vi"("1字节?"=FALSE, "数值"=w13181, "分辨率"=0.1) -> ("低字节"=w13183:dbl, "高字节1"=w13184:dbl)  [unwired: 2 in, 5 out]
                  }
                  frame Enabled {
                    w13187 = 255 ("高字节1")
                  }
                }
                n5047 = Build Array(w13180, w13179) -> (w13178:i32[])
              }
              frame 2 {
                # "最大允许充电电流"
                n5048 = disable-structure shown="启用" {
                  disable-tunnel: [w13196 w13199] -> w13191
                  disable-tunnel: [w13195 w13199] -> w13190
                  disable-tunnel: w13188 -> [w13193 _]
                  frame Disabled {
                    n5049 = Unbundle By Name(w13193) -> ("最大允许充电电流"=w13192:dbl)
                    n5050 = call "输入分辨率计算-EV05.vi"("1字节?"=FALSE, "数值"=w13192, "偏移量"=-3000.0, "分辨率"=0.1) -> ("低字节"=w13195:dbl, "高字节1"=w13196:dbl)  [unwired: 1 in, 5 out]
                  }
                  frame Enabled {
                    w13199 = 255 ("高字节1")
                  }
                }
                n5051 = Build Array(w13191, w13190) -> (w13189:i32[])
              }
              frame 3 {
                # "最小允许充电温度"
                n5052 = disable-structure shown="启用" {
                  disable-tunnel: [w13206 255 ("高字节1")] -> w13202
                  disable-tunnel: w13200 -> [w13204 _]
                  frame Disabled {
                    n5053 = Unbundle By Name(w13204) -> ("最小允许温度"=w13203:dbl)
                    n5054 = call "输入分辨率计算-EV05.vi"("1字节?"=TRUE, "数值"=w13203, "偏移量"=-40.0, "分辨率"=1.0) -> ("高字节1"=w13206:dbl)  [unwired: 1 in, 6 out]
                  }
                  frame Enabled {
                  }
                }
                n5055 = Build Array(w13202) -> (w13201:i32[])
              }
              frame 4 {
                # "最小充电电流"
                n5056 = disable-structure shown="启用" {
                  disable-tunnel: [w13217 w13220] -> w13213
                  disable-tunnel: [w13216 w13220] -> w13211
                  disable-tunnel: w13210 -> [w13215 _]
                  frame Disabled {
                    n5057 = Unbundle By Name(w13215) -> ("最小充电电流"=w13214:dbl)
                    n5058 = call "输入分辨率计算-EV05.vi"("1字节?"=FALSE, "数值"=w13214, "分辨率"=0.1) -> ("低字节"=w13216:dbl, "高字节1"=w13217:dbl)  [unwired: 2 in, 5 out]
                  }
                  frame Enabled {
                    w13220 = 255 ("高字节1")
                  }
                }
                n5059 = Build Array(w13213, w13211) -> (w13212:i32[])
              }
              frame 5 {
                # "电流步长"
                n5060 = disable-structure shown="启用" {
                  disable-tunnel: [w13229 w13232] -> w13224
                  disable-tunnel: [w13227 w13232] -> w13222
                  disable-tunnel: w13221 -> [w13226 _]
                  frame Disabled {
                    n5061 = Unbundle By Name(w13226) -> ("电流步长"=w13225:dbl)
                    n5062 = call "输入分辨率计算-EV05.vi"("1字节?"=FALSE, "数值"=w13225, "偏移量"=0.0, "分辨率"=1.0) -> ("低字节"=w13227:dbl, "高字节1"=w13229:dbl)  [unwired: 1 in, 5 out]
                  }
                  frame Enabled {
                    w13232 = 255 ("高字节1")
                  }
                }
                n5063 = Build Array(w13224, w13222) -> (w13223:i32[])
              }
              frame 6 {
                # "最小允许单体电压"
                n5064 = disable-structure shown="启用" {
                  disable-tunnel: [w13240 w13243] -> w13236
                  disable-tunnel: [w13239 w13243] -> w13234
                  disable-tunnel: w13233 -> [w13238 _]
                  frame Disabled {
                    n5065 = Unbundle By Name(w13238) -> ("最小允许单体电压"=w13237:dbl)
                    n5066 = call "输入分辨率计算-EV05.vi"("1字节?"=FALSE, "数值"=w13237, "分辨率"=0.001) -> ("低字节"=w13239:dbl, "高字节1"=w13240:dbl)  [unwired: 2 in, 5 out]
                  }
                  frame Enabled {
                    w13243 = 255 ("高字节1")
                  }
                }
                n5067 = Build Array(w13236, w13234) -> (w13235:i32[])
              }
              frame 7 {
                # "最大允许充电温度"
                n5068 = disable-structure shown="启用" {
                  disable-tunnel: [w13250 255 ("高字节1")] -> w13246
                  disable-tunnel: w13244 -> [w13248 _]
                  frame Disabled {
                    n5069 = Unbundle By Name(w13248) -> ("最大允许充电温度"=w13247:dbl)
                    n5070 = call "输入分辨率计算-EV05.vi"("1字节?"=TRUE, "数值"=w13247, "偏移量"=-40.0, "分辨率"=1.0) -> ("高字节1"=w13250:dbl)  [unwired: 1 in, 6 out]
                  }
                  frame Enabled {
                  }
                }
                n5071 = Build Array(w13246) -> (w13245:i32[])
              }
            }
            n5072 = Insert Into Array(array=w13161, new element=w13162) -> (w13165:dbl[])  [unwired: 1 in]
          }
          n5073 = Build Array(w13157) -> (w13159:dbl[][])
        }
        frame "最大允许总电压" {
          n5074 = Unbundle By Name(w13257) -> ("充电控制参数"=w13258:refnum<vi>)
          n5075 = property class="Clust (严格)"(reference=w13258) -> ("Value"=w13256:T6)  [unwired: 1 in, 2 out]
          n5076 = for {
            N: 8 -> [_]
            tunnel: w13256 -> [w13268]
            shift-right: [w13270] -> w13262
            shift-left: dbl[] [] -> [w13266]
            i -> [w13269]
            n5077 = case shown="1" w13269 {
              tunnel: w13268 -> [w13271 w13282 w13293 w13305 w13315 w13326 w13338 w13349]
              tunnel: [w13272 w13283 w13294 w13306 w13317 w13328 w13340 w13350] -> w13267
              frame 0, Default {
                # "最大允许单体电压"
                n5078 = disable-structure shown="启用" {
                  disable-tunnel: [w13278 w13281] -> w13274
                  disable-tunnel: [w13277 w13281] -> w13273
                  disable-tunnel: w13271 -> [w13276 _]
                  frame Disabled {
                    n5079 = Unbundle By Name(w13276) -> ("最大允许单体电压"=w13275:dbl)
                    n5080 = call "输入分辨率计算-EV05.vi"("1字节?"=FALSE, "数值"=w13275, "分辨率"=0.001) -> ("低字节"=w13277:dbl, "高字节1"=w13278:dbl)  [unwired: 2 in, 5 out]
                  }
                  frame Enabled {
                    w13281 = 255 ("高字节1")
                  }
                }
                n5081 = Build Array(w13274, w13273) -> (w13272:i32[])
              }
              frame 1 {
                # "最大允许总电压"
                n5082 = disable-structure shown="启用" {
                  disable-tunnel: [w13289 w13292] -> w13285
                  disable-tunnel: [w13288 w13292] -> w13284
                  disable-tunnel: w13282 -> [w13287 _]
                  frame Enabled {
                    n5083 = Unbundle By Name(w13287) -> ("最大允许总电压"=w13286:dbl)
                    n5084 = call "输入分辨率计算-EV05.vi"("1字节?"=FALSE, "数值"=w13286, "分辨率"=0.1) -> ("低字节"=w13288:dbl, "高字节1"=w13289:dbl)  [unwired: 2 in, 5 out]
                  }
                  frame Disabled {
                    w13292 = 255 ("高字节1")
                  }
                }
                n5085 = Build Array(w13285, w13284) -> (w13283:dbl[])
              }
              frame 2 {
                # "最大允许充电电流"
                n5086 = disable-structure shown="启用" {
                  disable-tunnel: [w13301 w13304] -> w13296
                  disable-tunnel: [w13300 w13304] -> w13295
                  disable-tunnel: w13293 -> [w13298 _]
                  frame Disabled {
                    n5087 = Unbundle By Name(w13298) -> ("最大允许充电电流"=w13297:dbl)
                    n5088 = call "输入分辨率计算-EV05.vi"("1字节?"=FALSE, "数值"=w13297, "偏移量"=-3000.0, "分辨率"=0.1) -> ("低字节"=w13300:dbl, "高字节1"=w13301:dbl)  [unwired: 1 in, 5 out]
                  }
                  frame Enabled {
                    w13304 = 255 ("高字节1")
                  }
                }
                n5089 = Build Array(w13296, w13295) -> (w13294:i32[])
              }
              frame 3 {
                # "最小允许充电温度"
                n5090 = disable-structure shown="启用" {
                  disable-tunnel: [w13311 255 ("高字节1")] -> w13307
                  disable-tunnel: w13305 -> [w13309 _]
                  frame Disabled {
                    n5091 = Unbundle By Name(w13309) -> ("最小允许温度"=w13308:dbl)
                    n5092 = call "输入分辨率计算-EV05.vi"("1字节?"=TRUE, "数值"=w13308, "偏移量"=-40.0, "分辨率"=1.0) -> ("高字节1"=w13311:dbl)  [unwired: 1 in, 6 out]
                  }
                  frame Enabled {
                  }
                }
                n5093 = Build Array(w13307) -> (w13306:i32[])
              }
              frame 4 {
                # "最小充电电流"
                n5094 = disable-structure shown="启用" {
                  disable-tunnel: [w13322 w13325] -> w13318
                  disable-tunnel: [w13321 w13325] -> w13316
                  disable-tunnel: w13315 -> [w13320 _]
                  frame Disabled {
                    n5095 = Unbundle By Name(w13320) -> ("最小充电电流"=w13319:dbl)
                    n5096 = call "输入分辨率计算-EV05.vi"("1字节?"=FALSE, "数值"=w13319, "分辨率"=0.1) -> ("低字节"=w13321:dbl, "高字节1"=w13322:dbl)  [unwired: 2 in, 5 out]
                  }
                  frame Enabled {
                    w13325 = 255 ("高字节1")
                  }
                }
                n5097 = Build Array(w13318, w13316) -> (w13317:i32[])
              }
              frame 5 {
                # "电流步长"
                n5098 = disable-structure shown="启用" {
                  disable-tunnel: [w13334 w13337] -> w13329
                  disable-tunnel: [w13332 w13337] -> w13327
                  disable-tunnel: w13326 -> [w13331 _]
                  frame Disabled {
                    n5099 = Unbundle By Name(w13331) -> ("电流步长"=w13330:dbl)
                    n5100 = call "输入分辨率计算-EV05.vi"("1字节?"=FALSE, "数值"=w13330, "偏移量"=0.0, "分辨率"=1.0) -> ("低字节"=w13332:dbl, "高字节1"=w13334:dbl)  [unwired: 1 in, 5 out]
                  }
                  frame Enabled {
                    w13337 = 255 ("高字节1")
                  }
                }
                n5101 = Build Array(w13329, w13327) -> (w13328:i32[])
              }
              frame 6 {
                # "最小允许单体电压"
                n5102 = disable-structure shown="启用" {
                  disable-tunnel: [w13345 w13348] -> w13341
                  disable-tunnel: [w13344 w13348] -> w13339
                  disable-tunnel: w13338 -> [w13343 _]
                  frame Disabled {
                    n5103 = Unbundle By Name(w13343) -> ("最小允许单体电压"=w13342:dbl)
                    n5104 = call "输入分辨率计算-EV05.vi"("1字节?"=FALSE, "数值"=w13342, "分辨率"=0.001) -> ("低字节"=w13344:dbl, "高字节1"=w13345:dbl)  [unwired: 2 in, 5 out]
                  }
                  frame Enabled {
                    w13348 = 255 ("高字节1")
                  }
                }
                n5105 = Build Array(w13341, w13339) -> (w13340:i32[])
              }
              frame 7 {
                # "最大允许充电温度"
                n5106 = disable-structure shown="启用" {
                  disable-tunnel: [w13355 255 ("高字节1")] -> w13351
                  disable-tunnel: w13349 -> [w13353 _]
                  frame Disabled {
                    n5107 = Unbundle By Name(w13353) -> ("最大允许充电温度"=w13352:dbl)
                    n5108 = call "输入分辨率计算-EV05.vi"("1字节?"=TRUE, "数值"=w13352, "偏移量"=-40.0, "分辨率"=1.0) -> ("高字节1"=w13355:dbl)  [unwired: 1 in, 6 out]
                  }
                  frame Enabled {
                  }
                }
                n5109 = Build Array(w13351) -> (w13350:i32[])
              }
            }
            n5110 = Insert Into Array(array=w13266, new element=w13267) -> (w13270:dbl[])  [unwired: 1 in]
          }
          n5111 = Build Array(w13262) -> (w13264:dbl[][])
        }
        frame "最大允许充电电流" {
          n5112 = Unbundle By Name(w13362) -> ("充电控制参数"=w13363:refnum<vi>)
          n5113 = property class="Clust (严格)"(reference=w13363) -> ("Value"=w13361:T6)  [unwired: 1 in, 2 out]
          n5114 = for {
            N: 8 -> [_]
            tunnel: w13361 -> [w13373]
